vi "Read Purge.vi"(8 "error in (no error)":errorcluster, 11 "Potting Procedure in":refnum<class "Potting Procedure.lvclass">) -> (0 "error out":errorcluster, 2 "Purge":T1, 3 "Potting Procedure out":refnum<class "Potting Procedure.lvclass">)   [LabVIEW 2011, in "Potting Procedure.lvclass"]
uses:
  Potting Procedure.lvclass
  Type Definitions/Purge.ctl
  Potting Procedure.lvclass/Potting Procedure.ctl
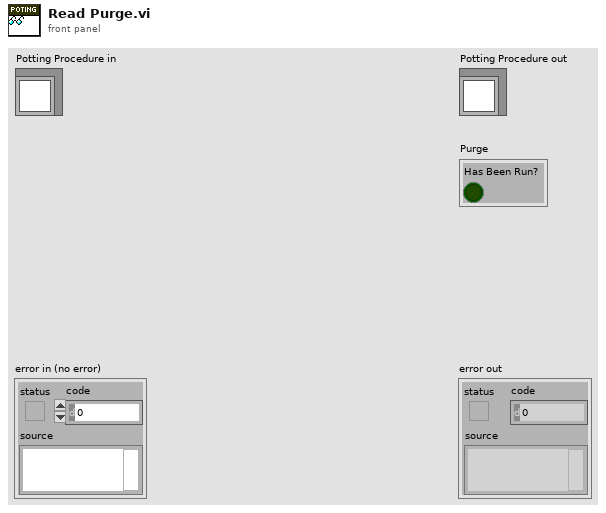
[diagram p1: front panel]
types:
  T1 = typedef "Purge.ctl" = cluster{"Has Been Run?":bool}
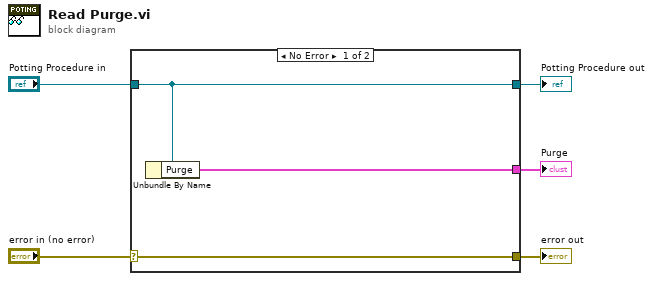
[diagram p0: block diagram]
diagram:
  n1 = case shown="No Error" "error in (no error)" {
    selector: "error in (no error)" -> [w8 w9]
    tunnel: [w8 w9] -> w4
    tunnel: [w7 w10] -> w2
    tunnel: "Potting Procedure in" -> [w7 w10]
    tunnel: [w6 _] -> w1
    frame No Error {
      n2 = Unbundle By Name(w7) -> ("Purge"=w6:T1)
    }
    frame Error {
    }
  }
  "error out" <- w4
  "Potting Procedure out" <- w2
  "Purge" <- w1
